vi "Vision Processing.vi"(4 "error in (no error)":errorcluster) -> ()   [LabVIEW 2013]
doc: "This VI runs in parallel to other tasks. It gets images from the camera, processes them for color or shape and use that information to affect robot behavior."
uses:
  <vilib>/Rock Robotics/WPI/Camera/WPI_CameraImageSize.ctl
  Vision/TargetType.ctl
  Robot Global Data.vi
panel:
  in  "Score Limit 2":dbl=80.0
  in  "Image Size 2":T1=enum."320x240"
  in  "Color Components 2":T2={"Hue"={108.0, 140.0}, "Sat"={97.0, 255.0}, "Val"={178.0, 255.0}} {"Val" scale=0.0..255.0; "Sat" scale=0.0..255.0; "Hue" scale=0.0..255.0 scale format="%#_3g"}
  out "Hot 2":bool
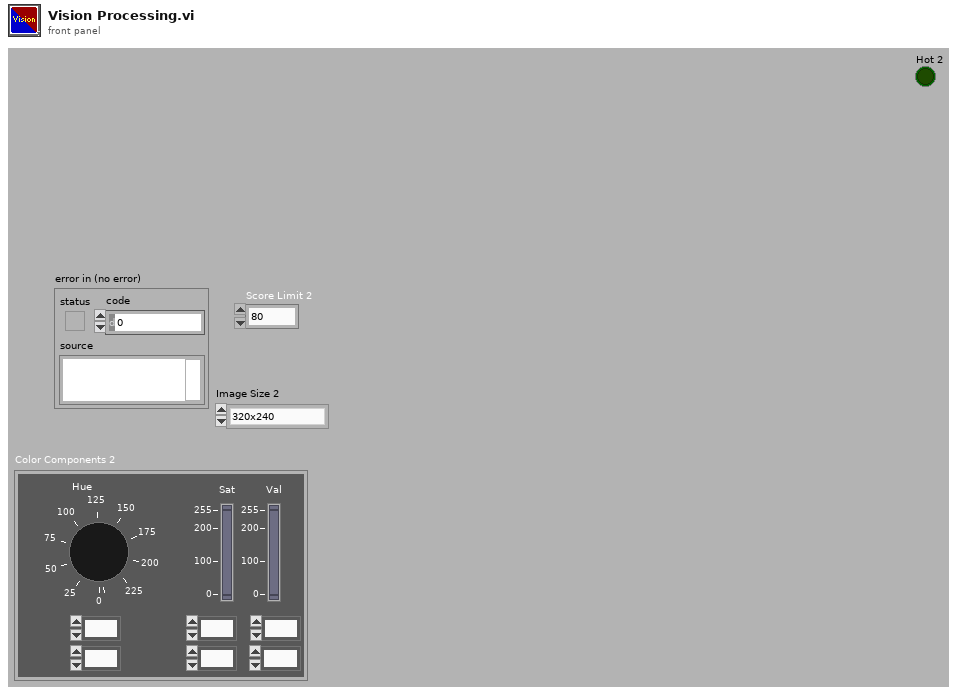
[diagram p1: front panel]
types:
  T1 = typedef "WPI_CameraImageSize.ctl" = enum16{"640x480", "320x240", "160x120"}
  T2 = cluster{"Hue":cluster{dbl, dbl}, "Sat":cluster{dbl, dbl}, "Val":cluster{dbl, dbl}}
  T3 = typedef "Image Type" = u32
  T4 = typedef "WPI_CameraDevRef.ctl" = cluster{"Camera Address":string, "CameraStatus":errorcluster, "Acquire Image Notifier":refnum<notifier>}
  T5 = typedef "IMAQ Image.ctl" = refnum<image>
  T6 = typedef "TargetType.ctl" = enum16{"Not Hot", "Hot"}
  T7 = cluster{"Horizontal":bool, "Aspect Score":dbl, "Rect Score":dbl, cluster{"Left":dbl, "Top":dbl, "Right":dbl, "Bottom":dbl}, "Equiv H":dbl, "Equiv V":dbl}[]
  T8 = cluster{"Scores":cluster{"Total":dbl, "Left":dbl, "Right":dbl, "Ratio":dbl, "Vertical":dbl, "index":i32, "State":T6}, "Verticals":cluster{"Horizontal?":bool, "Aspect Score":dbl, "Rect Score":dbl, cluster{"Left":dbl, "Top":dbl, "Right":dbl, "Bottom":dbl}, "Equiv H":dbl, "Equiv V":dbl}, "Horizontals":cluster{"Horizontal?":bool, "Aspect Score":dbl, "Rect Score":dbl, cluster{"Left":dbl, "Top":dbl, "Right":dbl, "Bottom":dbl}, "Equiv H":dbl, "Equiv V":dbl}, "Validated":bool}[]
  T9 = cluster{"Scores":cluster{"Total":dbl, "Left":dbl, "Right":dbl, "Ratio":dbl, "Vertical":dbl, "index":i32, "State":T6}, "Verticals":cluster{"Horizontal?":bool, "Aspect Score":dbl, "Rect Score":dbl, cluster{"Left":dbl, "Top":dbl, "Right":dbl, "Bottom":dbl}, "Equiv H":dbl, "Equiv V":dbl}, "Horizontals":cluster{"Horizontal?":bool, "Aspect Score":dbl, "Rect Score":dbl, cluster{"Left":dbl, "Top":dbl, "Right":dbl, "Bottom":dbl}, "Equiv H":dbl, "Equiv V":dbl}, "Validated":bool}
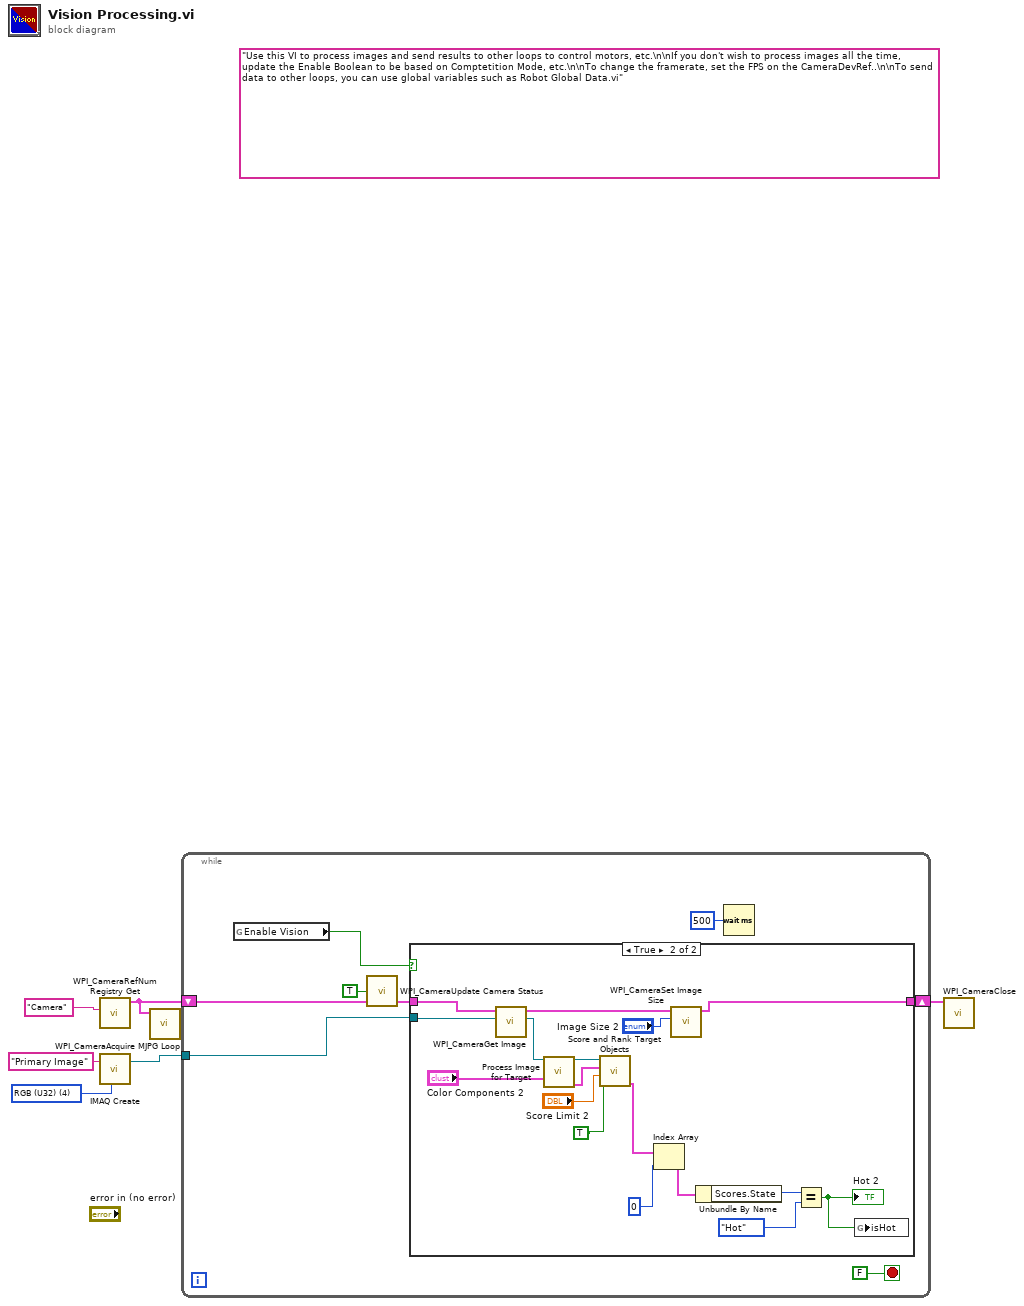
[diagram p0: block diagram]
diagram:
  w6 = T3 4 items=["Grayscale (U8)", "Grayscale (I16)", "Grayscale (SGL)", "Complex (CSG)", "RGB (U32)", "HSL (U32)", "RGB (U64)"] ("Image Type")
  (unwired) "Use this VI to process images and send results to other loops to control motors, etc.\n\nIf you don't wish to process images all the time, update the Enable Boolean to be based on Comptetition Mode, etc.\n\nTo change the framerate, set the FPS on the CameraDevRef..\n\nTo send data to other loops, you can use global variables such as Robot Global Data.vi"
  n1 = call <vilib>:"WPI_CameraRefNum Registry Get.vi"("refnum name"="Camera") -> ("CameraDevRef"=w2:T4)  [unwired: 9 in, 1 out]
  n2 = call "IMAQ Create"("Image Name"="Primary Image", "Image Type"=w6) -> ("New Image"=w4:T5)  [unwired: 2 in, 2 out]
  n3 = call <vilib>:"WPI_CameraAcquire MJPG Loop.vi"("CameraDevRef"=w2) -> ()  [unwired: 11 in]
  n4 = while {
    tunnel: w4 -> [w14]
    shift-right: [w13] -> w3
    shift-left: w2 -> [w12]
    stop <- FALSE stop-if-true
    n5 = global read "Robot Global Data.vi" "Enable Vision"() -> (w9:bool)
    n6 = call <vilib>:"WPI_CameraUpdate Camera Status.vi"("CameraDevRef In"=w12, "Enable Vision"=TRUE) -> ("CameraDevRef Out"=w11:T4)  [unwired: 3 in]
    n7 = case shown="True" w9 {
      tunnel: w14 -> [_ w31]
      tunnel: [w15 w32] -> w13
      tunnel: w11 -> [w15 w30]
      frame False {
      }
      frame True {
        n8 = call <vilib>:"WPI_CameraGet Image.vi"("Image"=w31, "CameraDevRef"=w30) -> ("Image Out"=w28:T5, "CameraDevRef Out"=w29:T4)  [unwired: 1 in, 7 out]
        n9 = call "Process Image for Target.vi"("Src Image"=w28, "Color Components"="Color Components 2") -> ("Src Image Out"=w27:T5, "Particles"=w26:T7)  [unwired: 11 in, 1 out]
        n10 = call "Score and Rank Target Objects.vi"("Annotate"=TRUE, "Score Limit"="Score Limit 2", "Particles"=w26, "Image in"=w27) -> ("Target Info"=w22:T8)  [unwired: 6 in, 1 out]
        n11 = Index Array(array=w22, index=0) -> (element=w20:T9)
        n12 = call <vilib>:"WPI_CameraSet Image Size.vi"("Image Size"="Image Size 2", "CameraDevRef"=w29) -> ("CameraDevRef Out"=w32:T4)  [unwired: 1 in, 8 out]
        n13 = Unbundle By Name(w20) -> ("Scores.State"=w19:T6)
        n14 = Equal?(x=w19, y=TargetType."Hot" ("Scores.State")) -> (x = y?=w17:bool)
        "Hot 2" <- w17
        n15 = global write "Robot Global Data.vi" "isHot"(w17) -> ()
      }
    }
    n16 = Wait (ms)(milliseconds to wait=u32 500) -> ()  [unwired: 1 out]
  }
  n17 = call <vilib>:"WPI_CameraClose.vi"("CameraDevRef"=w3) -> ()  [unwired: 1 in, 10 out]
